vi "PC_Shot_Calculations_Overlay (DONE).vi"(5 "Table Walls Input":sgl[](array[numeric]), 7 "Player and Puck Input":T1, 8 "Error  In":errorcluster, 10 "Shot Inputs":cluster{"Bounce":dbl[][], "Straight":dbl[][]}, 11 "Image In":T2) -> (0 "Error Out":errorcluster, 2 "Shot Outputs (Pass Through)":cluster{"Bounce":dbl[][], "Straight":dbl[][]}, 3 "Image Out":T2)   [LabVIEW 2017]
uses:
  <vilib>/vision/Image Controls.llb/IMAQ Image.ctl
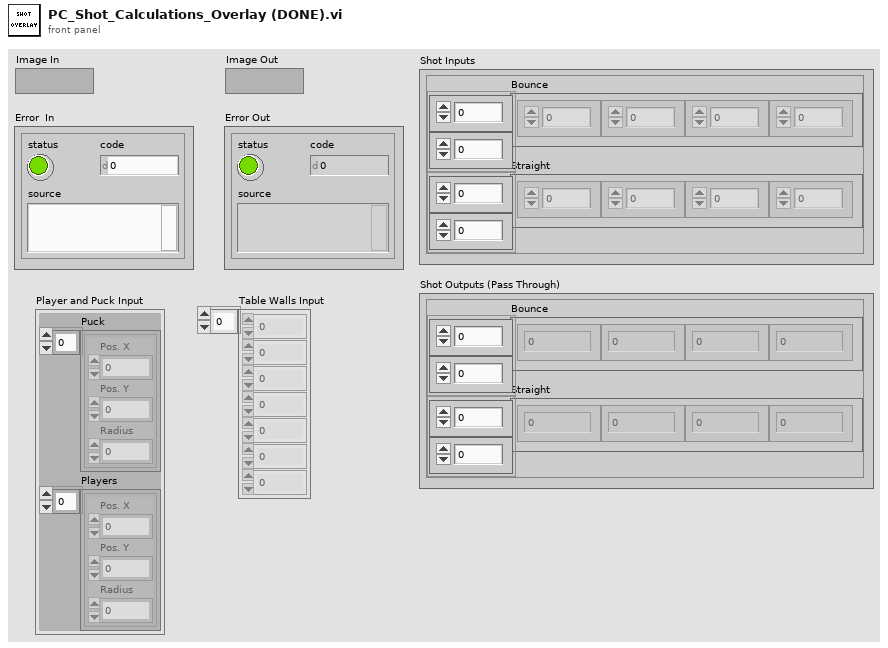
[diagram p1: front panel]
types:
  T1 = cluster{"Puck":cluster{"Pos. X":i32, "Pos. Y":i32, "Radius":i32}[], "Players":cluster{"Pos. X":i32, "Pos. Y":i32, "Radius":i32}[]}
  T2 = typedef "IMAQ Image.ctl" = refnum<image>
  T3 = cluster{"Pos. X":i32, "Pos. Y":i32, "Radius":i32}[]
  T4 = cluster{"Pos. X":i32, "Pos. Y":i32, "Radius":i32}
  T5 = cluster{"Numeric Control":sgl, "Numeric Control":dbl}
  T6 = cluster{"Numeric Control":dbl, "Numeric Control":sgl}
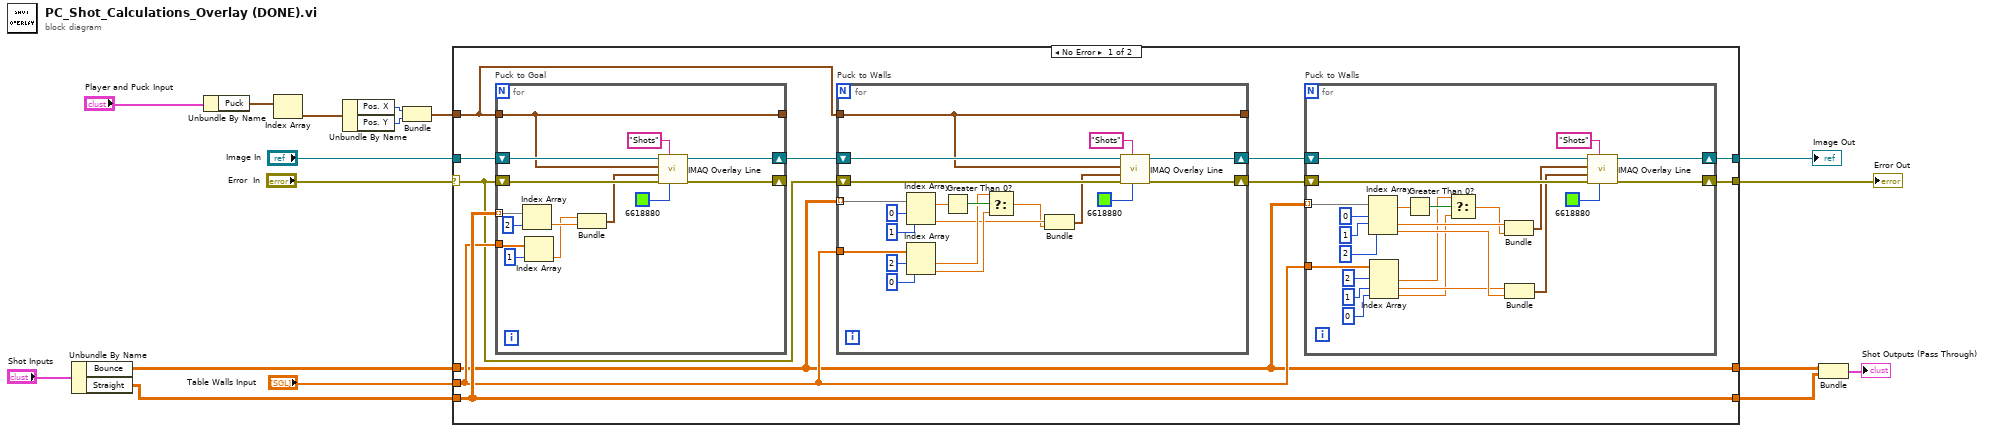
[diagram p0: block diagram]
diagram:
  n1 = Unbundle By Name("Shot Inputs") -> ("Bounce"=w5:dbl[][], "Straight"=w4:dbl[][])
  n2 = Unbundle By Name("Player and Puck Input") -> ("Puck"=w16:T3)
  n3 = Index Array(array=w16) -> (element=w15:T4)  [unwired: 1 in]
  n4 = Unbundle By Name(w15) -> ("Pos. X"=w13:i32, "Pos. Y"=w12:i32)
  n5 = Bundle("Pos. X"=w13, "Pos. Y"=w12) -> (w11:cluster{"Pos. X":i32, "Pos. Y":i32})  [unwired: 1 in]
  n6 = case shown="No Error" "Error  In" {
    selector: "Error  In" -> [w19 w90]
    tunnel: "Image In" -> [w28 w89]
    tunnel: w11 -> [w18 _]
    tunnel: w4 -> [w22 w87]
    tunnel: w5 -> [w20 w88]
    tunnel: "Table Walls Input" -> [w21 _]
    tunnel: [w24 w89] -> w9
    tunnel: [w23 w90] -> w8
    tunnel: [w22 w87] -> w1
    tunnel: [w20 w88] -> w2
    frame No Error {
      n7 = for "Puck to Goal" {
        shift-right: [w62] -> w27
        shift-left: w28 -> [w61]
        shift-right: [w60] -> _
        shift-left: w19 -> [w59]
        tunnel: w21 -> [w56]
        tunnel: w18 -> [w55]
        tunnel: [w55] -> _
        tunnel: w22 -> [w53] mode=indexing
        n8 = Index Array(array=w53, index=2) -> (element=w51:dbl)
        n9 = Index Array(array=w56, index=1) -> (element=w50:sgl)
        n10 = Bundle("Numeric Control"=w50, "Numeric Control"=w51) -> (w49:T5)  [unwired: 1 in]
        n11 = call "IMAQ Overlay Line"("Color"=u32 6618880, "Group"="Shots", "error in (no error)"=w59, "End Point"=w49, "Start Point"=w55, "Image"=w61) -> ("error out"=w60:errorcluster, "Image Out"=w62:T2)  [unwired: 4 in]
      }
      n12 = for "Puck to Walls" {
        shift-right: [w48] -> w26
        shift-left: w27 -> [w47]
        shift-right: [w46] -> w25
        shift-left: w19 -> [w45]
        tunnel: w21 -> [w37]
        tunnel: w18 -> [w42]
        tunnel: [w42] -> _
        tunnel: w20 -> [w41] mode=indexing
        n13 = Index Array(array=w41, index #1=0 ("index"), index #2=1 ("index")) -> (element #1=w38:dbl, element #2=w31:dbl)
        n14 = Index Array(array=w37, index #1=2 ("index"), index #2=0 ("index")) -> (element #1=w34:sgl, element #2=w33:sgl)
        n15 = Greater Than 0?(x=w38) -> (x > 0?=w39:bool)
        n16 = Select(t=w34, s=w39, f=w33) -> (s? t:f=w30:sgl)
        n17 = Bundle("Numeric Control"=w31, "Numeric Control"=w30) -> (w29:T6)  [unwired: 1 in]
        n18 = call "IMAQ Overlay Line"("Color"=u32 6618880, "Group"="Shots", "error in (no error)"=w45, "End Point"=w29, "Start Point"=w42, "Image"=w47) -> ("error out"=w46:errorcluster, "Image Out"=w48:T2)  [unwired: 4 in]
      }
      n19 = for "Puck to Walls" {
        shift-right: [w86] -> w24
        shift-left: w26 -> [w85]
        shift-right: [w84] -> w23
        shift-left: w25 -> [w83]
        tunnel: w20 -> [w76] mode=indexing
        tunnel: w21 -> [w73]
        n20 = Index Array(array=w76, index #1=0 ("index"), index #2=1 ("index"), index #3=2 ("index")) -> (element #1=w79:dbl, element #2=w72:dbl, element #3=w69:dbl)
        n21 = Index Array(array=w73, index #1=2 ("index"), index #2=1 ("index"), index #3=0 ("index")) -> (element #1=w67:sgl, element #2=w66:sgl, element #3=w65:sgl)
        n22 = Greater Than 0?(x=w79) -> (x > 0?=w78:bool)
        n23 = Select(t=w67, s=w78, f=w65) -> (s? t:f=w64:sgl)
        n24 = Bundle("Numeric Control"=w72, "Numeric Control"=w64) -> (w63:T6)  [unwired: 1 in]
        n25 = Bundle("Numeric Control"=w66, "Numeric Control"=w69) -> (w68:T5)  [unwired: 1 in]
        n26 = call "IMAQ Overlay Line"("Color"=u32 6618880, "Group"="Shots", "error in (no error)"=w83, "End Point"=w68, "Start Point"=w63, "Image"=w85) -> ("error out"=w84:errorcluster, "Image Out"=w86:T2)  [unwired: 4 in]
      }
    }
    frame Error {
    }
  }
  "Image Out" <- w9
  "Error Out" <- w8
  n27 = Bundle("Bounce"=w2, "Straight"=w1) -> (→"Shot Outputs (Pass Through)":cluster{"Bounce":dbl[][], "Straight":dbl[][]})  [unwired: 1 in]
